vi "dinamikyapıdabytebirleştirme.vi"() -> ()   [LabVIEW 2023]
panel:
  out "Array 8":u32[](array[numeric]) format="%02x"
  out "output array":bool[](array[boolean])
  out "Boolean array":bool[](array[boolean])
  in  "Array 6":cluster{"Boolean":bool, "Boolean 2":bool}[](array[cluster])
  # "4"
  # "4"
  # "4"
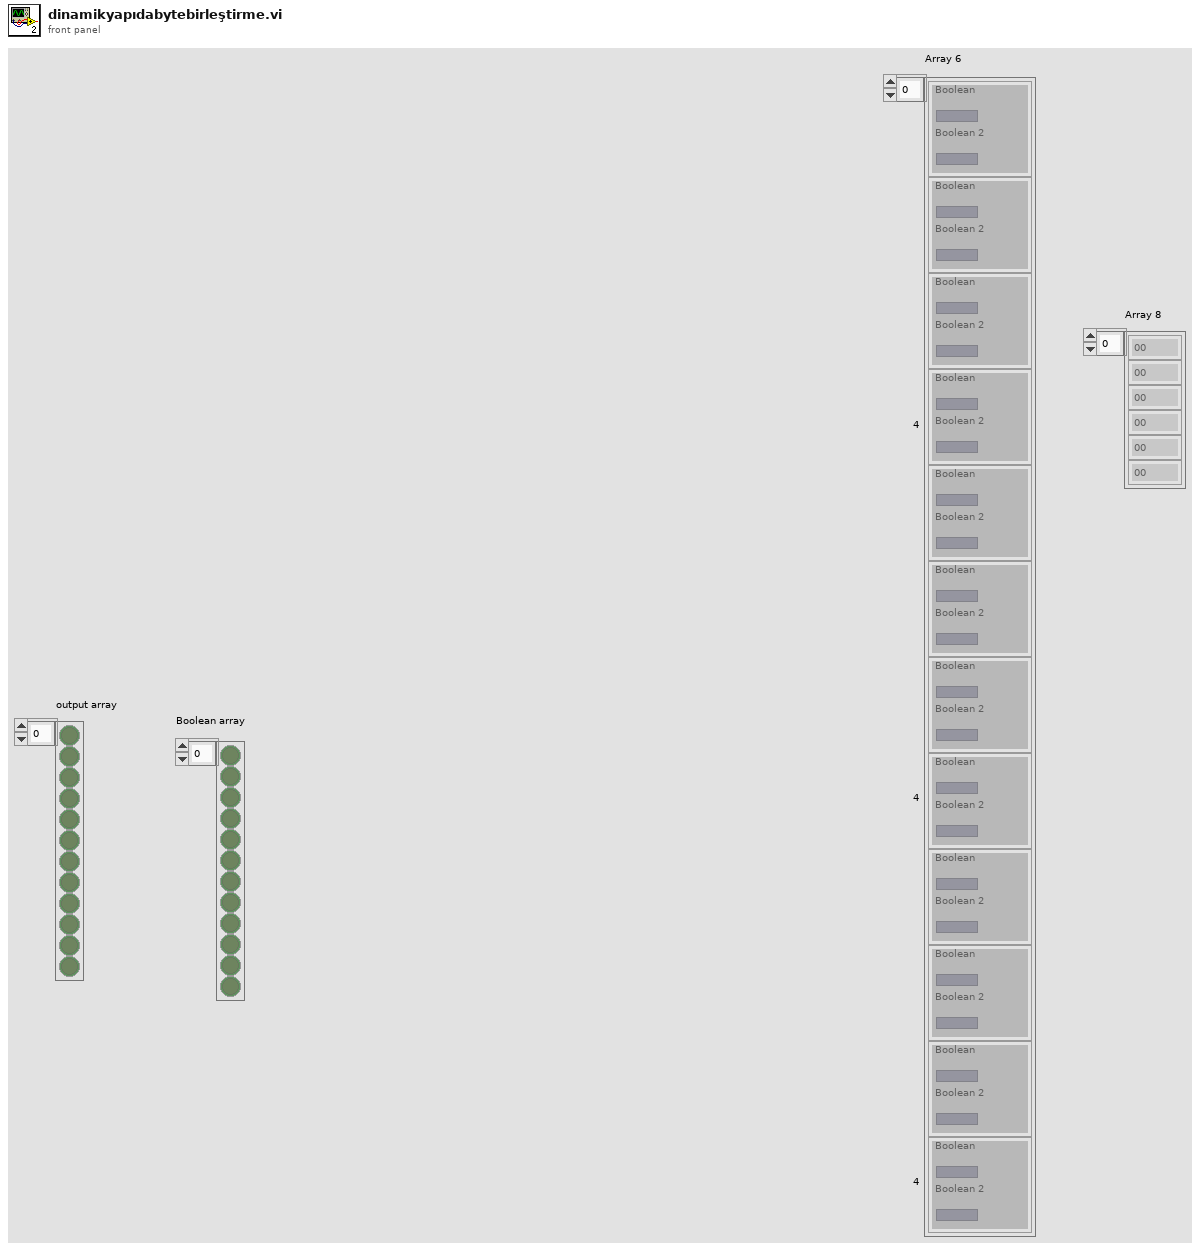
[diagram p1: front panel]
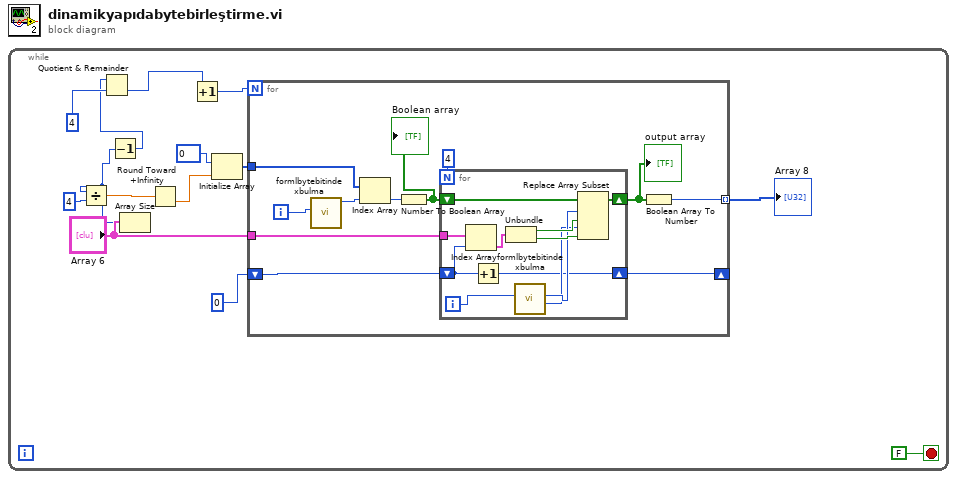
[diagram p0: block diagram]
diagram:
  n1 = while {
    stop <- FALSE stop-if-true
    n2 = Array Size(array="Array 6") -> (size(s)=w2:i32)
    n3 = Divide(x=w2, y=4) -> (x/y=w14:dbl)
    n4 = Decrement(x=w2) -> (x-1=w1:i32)
    n5 = Quotient & Remainder(x=w1, y=4 ("x")) -> (floor(x/y)=w5:i32)  [unwired: 1 out]
    n6 = Round Toward +Infinity(x=w14) -> (ceil(x): smallest int >= x=w3:dbl)
    n7 = Increment(x=w5) -> (x+1=w6:i32)
    n8 = Initialize Array(u8 0, w3) -> (w7:u8[])
    n9 = for {
      N: w6 -> [_]
      tunnel: "Array 6" -> [w24]
      tunnel: [w19] -> w11 mode=indexing
      shift-right: [w17] -> _
      shift-left: 0 -> [w15]
      tunnel: w7 -> [w16]
      i -> [w23]
      n10 = call "formlbytebitindexbulma.vi"("chanell -1"=w23) -> ("B"=w22:i32)  [unwired: 8 in, 2 out]
      n11 = Index Array(array=w16, index=w22) -> (element=w21:u8)
      n12 = Number To Boolean Array(number=w21) -> (Boolean array=w25:bool[])
      "Boolean array" <- w25
      n13 = for {
        N: 4 -> [_]
        tunnel: w24 -> [w30]
        shift-right: [w34] -> w20
        shift-left: w25 -> [w26]
        shift-right: [w27] -> w17
        shift-left: w15 -> [w28]
        i -> [w31]
        n14 = Index Array(array=w30, index=w28) -> (element=w29:cluster{"Boolean":bool, "Boolean 2":bool})
        n15 = Increment(x=w28) -> (x+1=w27:i32)
        n16 = Unbundle(w29) -> ("Boolean"=w36:bool, "Boolean 2"=w35:bool)
        n17 = call "formlbytebitindexbulma.vi"("chanell -1"=w31) -> ("bb"=w32:i32, "Bb"=w33:i32)  [unwired: 8 in, 1 out]
        n18 = Replace Array Subset(array=w26, new element #1=w36, index #1=w33, new element #2=w35, index #2=w32) -> (w34:bool[])
      }
      "output array" <- w20
      n19 = Boolean Array To Number(Boolean array=w20) -> (number=w19:u32)
    }
    "Array 8" <- w11
  }
